vi "GetCellInfo.vi"(8 "error in (no error)":errorcluster, 11 "SnakeBodyCell in":refnum<class "SnakeBodyCell.lvclass">) -> (0 "error out":errorcluster, 1 "Cell":T3, 2 "Color":u32, 3 "SnakeBodyCell out":refnum<class "SnakeBodyCell.lvclass">, 4 "CellPosInBody":u16, 5 "Direction":T4, 6 "Position":T2, 7 "DisplaySize":T1)   [LabVIEW 2018, in "SnakeBodyCell.lvclass"]
uses:
  SnakeBodyCell.lvclass
  Typedefs/UnitDirection.ctl
  Typedefs/CellType.ctl
  Typedefs/XYposition.ctl
  Typedefs/DisplaySize.ctl
  SnakeBodyCell.lvclass/SnakeBodyCell.ctl
panel:
  # "Connector Pane"
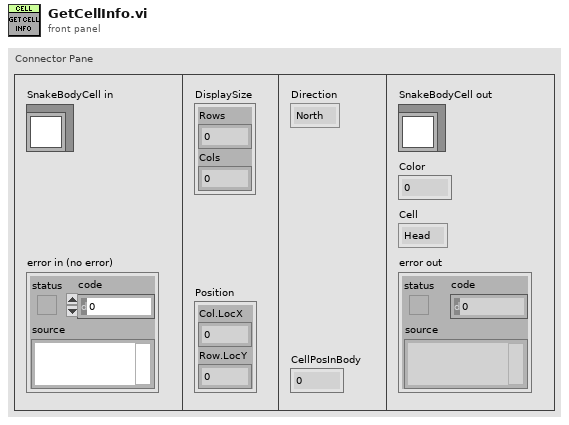
[diagram p1: front panel]
types:
  T1 = typedef "DisplaySize.ctl" = cluster{"Rows":i32, "Cols":i32}
  T2 = typedef "XYposition.ctl" = cluster{"Col.LocX":i32, "Row.LocY":i32}
  T3 = typedef "CellType.ctl" = enum16{"Head", "Tail", "Body"}
  T4 = typedef "UnitDirection.ctl" = enum16{"North", "East", "South", "West"}
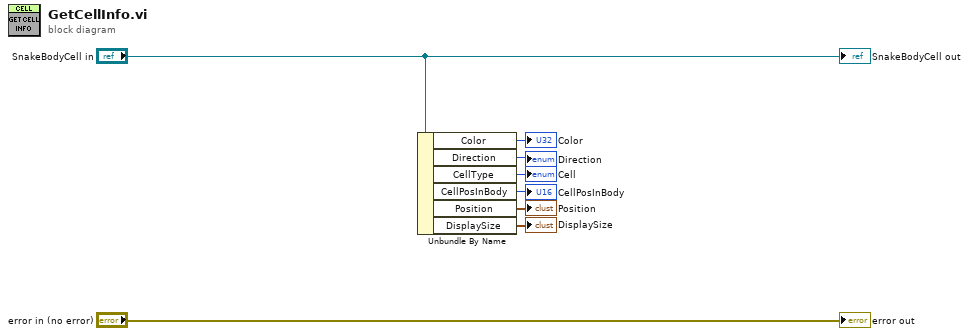
[diagram p0: block diagram]
diagram:
  n1 = Unbundle By Name("SnakeBodyCell in") -> ("Color"=→"Color":u32, "Direction"=→"Direction":T4, "CellType"=→"Cell":T3, "CellPosInBody"=→"CellPosInBody":u16, "Position"=→"Position":T2, "DisplaySize"=→"DisplaySize":T1)
  "error out" <- "error in (no error)"
  "SnakeBodyCell out" <- "SnakeBodyCell in"
